vi "TEST AMI 430.vi"() -> ()   [LabVIEW 2017]
uses:
  magneticField.ctl
  Status AMI.ctl
  AMI 430_Hardware_Module.ctl
  commsControl.ctl
panel:
  out "state X":T1=1 items=["Unknown", "RAMPING to target field/current", "HOLDING at the target field/current", "PAUSED", "Ramping in MANUAL UP mode", "Ramping in MANUAL DOWN mode", "ZEROING CURRENT (in progress)", "Quench detected", "At ZERO current", "Heating persistent switch", "Cooling persistent switch", "External Rampdown active"]
  out "state Y":T1=1 items=["Unknown", "RAMPING to target field/current", "HOLDING at the target field/current", "PAUSED", "Ramping in MANUAL UP mode", "Ramping in MANUAL DOWN mode", "ZEROING CURRENT (in progress)", "Quench detected", "At ZERO current", "Heating persistent switch", "Cooling persistent switch", "External Rampdown active"]
  out "state Z":T1=1 items=["Unknown", "RAMPING to target field/current", "HOLDING at the target field/current", "PAUSED", "Ramping in MANUAL UP mode", "Ramping in MANUAL DOWN mode", "ZEROING CURRENT (in progress)", "Quench detected", "At ZERO current", "Heating persistent switch", "Cooling persistent switch", "External Rampdown active"]
  out "Z field":dbl format="%.6f"
  out "Y field":dbl format="%.6f"
  out "X field":dbl format="%.6f"
  in  "RAMPING Z":bool
  in  "RAMPING Y":bool
  in  "RAMPING X":bool
  in  "SET X":bool
  in  "SET Z":bool
  in  "SET Y":bool
  in  "Settings X":T2={"magneticFieldUnits"=1, "rampRateUnits"=1, "rampRate"=0.0, "targetField"=0.0, "rampingMode"=1} {"rampingMode" items=["RAMP", "PAUSE", "MANUAL UP", "MANUAL DOWN", "ZERO"]; "targetField" format="%.3f"; "rampRate" format="%.3f"; "rampRateUnits" items=["Per SECOND", "Per MINUTE"]; "magneticFieldUnits" items=["KGauss", "Tesla"]}
  in  "Settings Z":T2={"magneticFieldUnits"=1, "rampRateUnits"=1, "rampRate"=0.0, "targetField"=0.0, "rampingMode"=1} {"rampingMode" items=["RAMP", "PAUSE", "MANUAL UP", "MANUAL DOWN", "ZERO"]; "targetField" format="%.3f"; "rampRate" format="%.3f"; "rampRateUnits" items=["Per SECOND", "Per MINUTE"]; "magneticFieldUnits" items=["KGauss", "Tesla"]}
  in  "Settings Y":T2={"magneticFieldUnits"=1, "rampRateUnits"=1, "rampRate"=0.0, "targetField"=0.0, "rampingMode"=1} {"rampingMode" items=["RAMP", "PAUSE", "MANUAL UP", "MANUAL DOWN", "ZERO"]; "targetField" format="%.3f"; "rampRate" format="%.3f"; "rampRateUnits" items=["Per SECOND", "Per MINUTE"]; "magneticFieldUnits" items=["KGauss", "Tesla"]}
  out "Waveform Chart":T3(graph)
  out "error out":errorcluster
  in  "stop":bool
  # "AMI 430 MAGNETIC FIELD SYSTEM TEST PANEL"
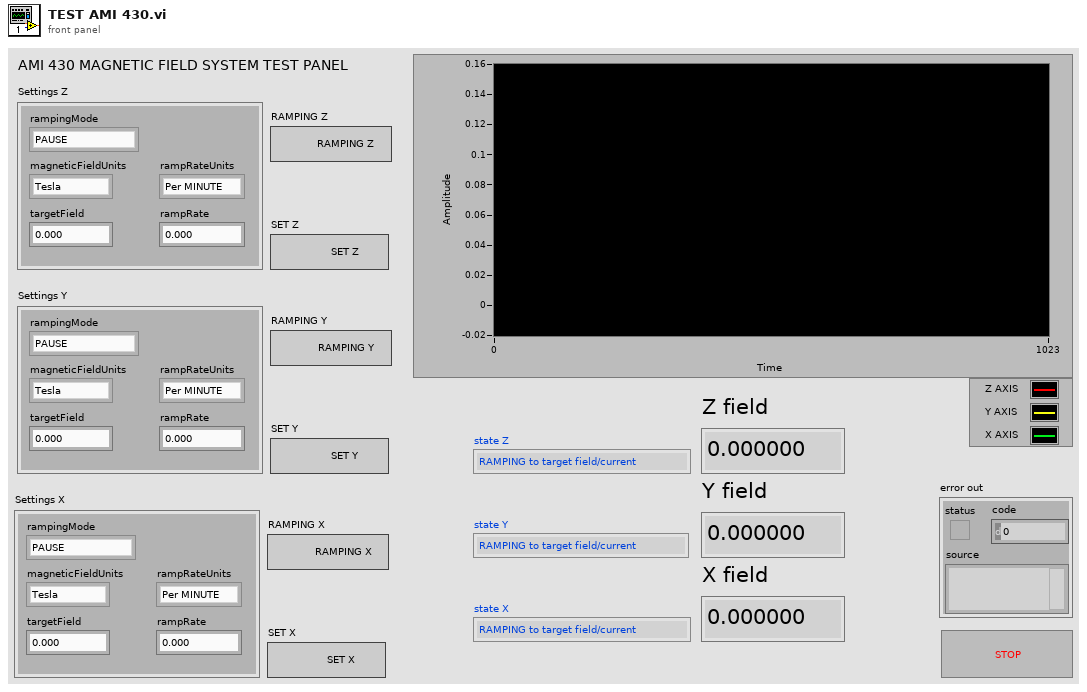
[diagram p1: front panel]
types:
  T1 = typedef "Status AMI.ctl" = u16
  T2 = typedef "magneticField.ctl" = cluster{"magneticFieldUnits":u16, "rampRateUnits":u16, "rampRate":dbl, "targetField":dbl, "rampingMode":u16}
  T3 = cluster{"magneticField":dbl, "magneticField":dbl, "magneticField":dbl}
  T4 = typedef "AMI 430_Hardware_Module.ctl" = enum16{"INICIALIZAR", "SET UNIDADES CAMPO", "SET UNIDADES RAMPA", "SET CAMPO", "SET  RAMPA", "SET RAMPING MODE", "READ CAMPO", "STATUS", "SHUTDOWN"}
  T5 = typedef "commsControl.ctl" = cluster{"connection ID":refnum<k5>, "IP":string, "Active Comm Interface":u16, "Serial Port":refnum<visa-resource-name>, "Programmer Type":u16, "connection ID":refnum<k5>, "output cluster":cluster{"GPIB address":i16, "GPIB bus":i16}}
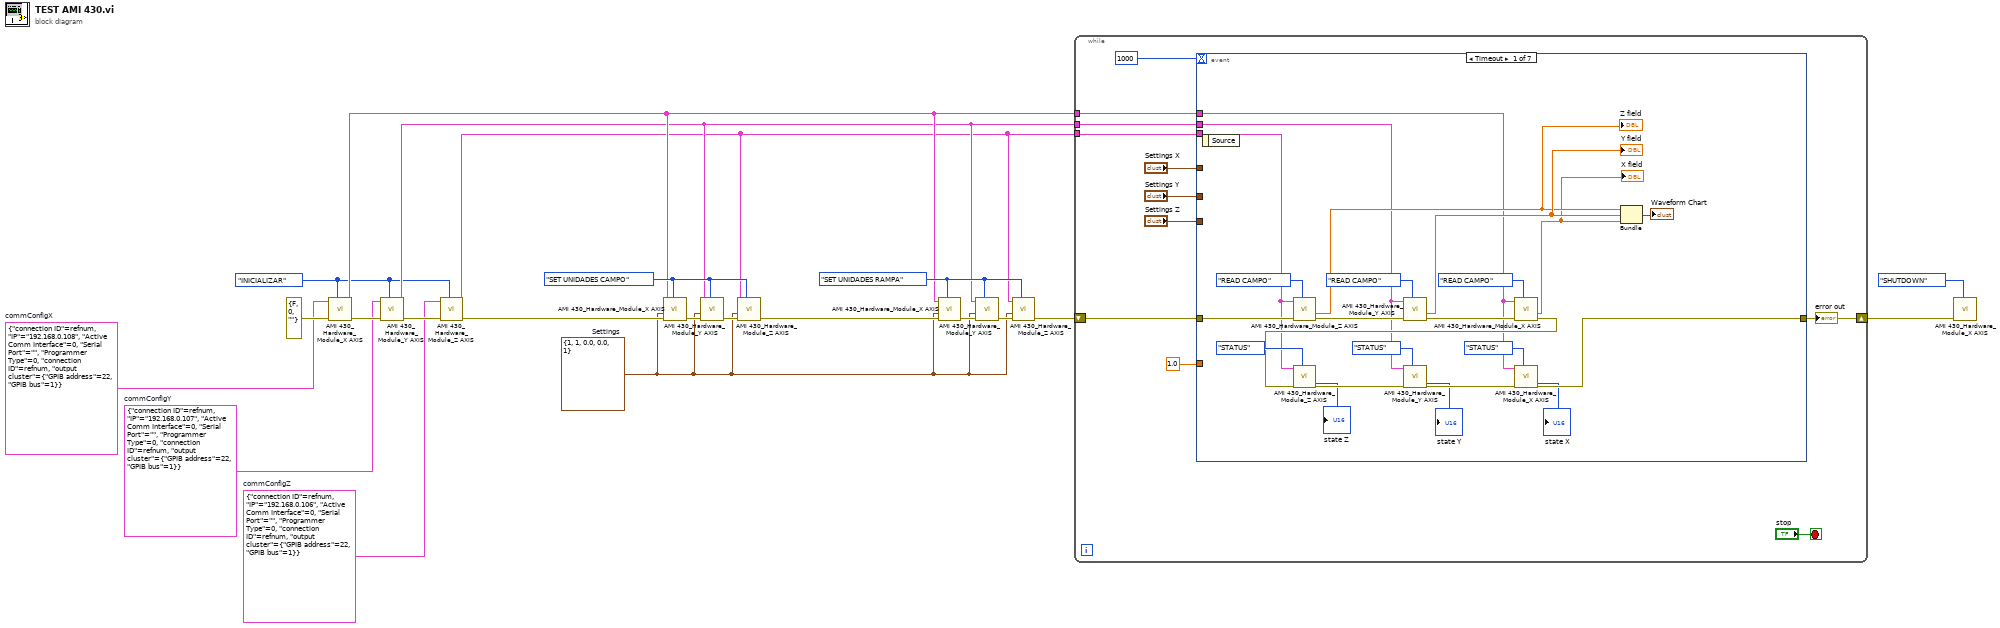
[diagram p0: block diagram]
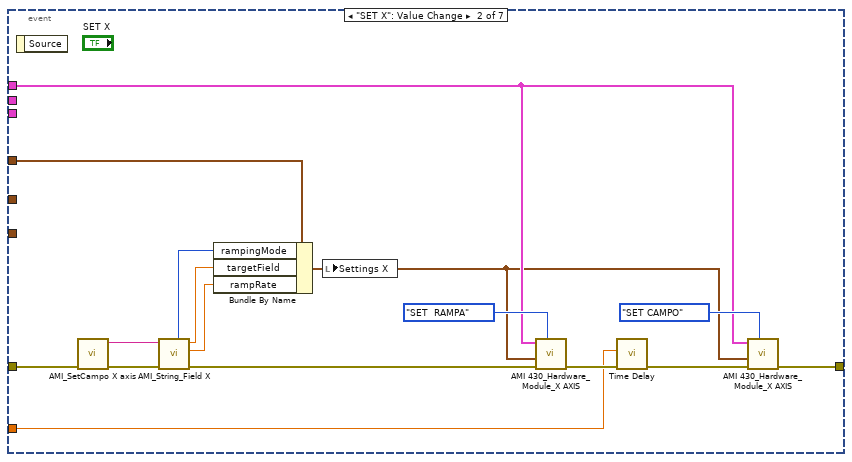
[diagram p2: hidden frame]
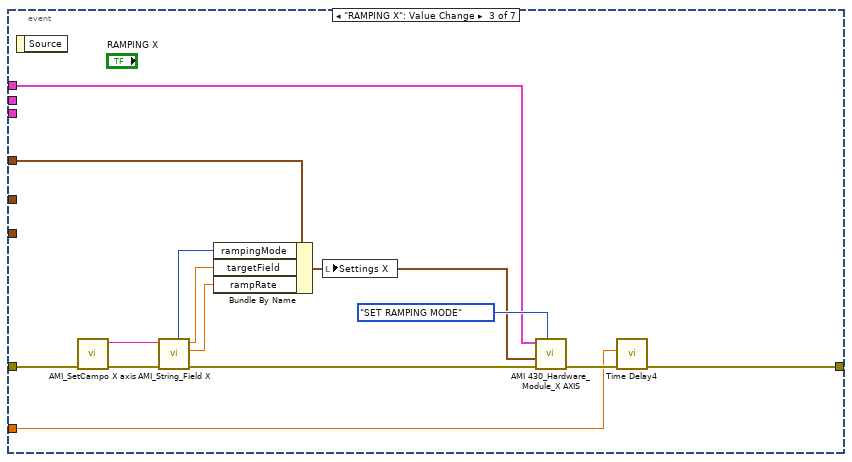
[diagram p3: hidden frame]
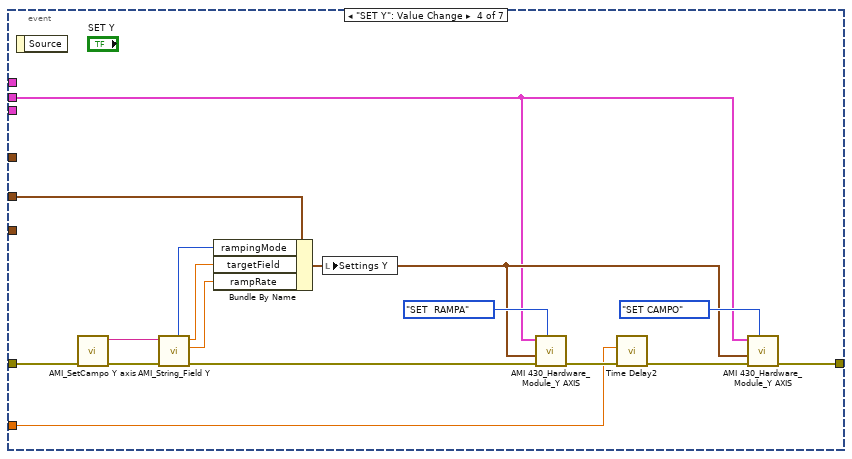
[diagram p4: hidden frame]
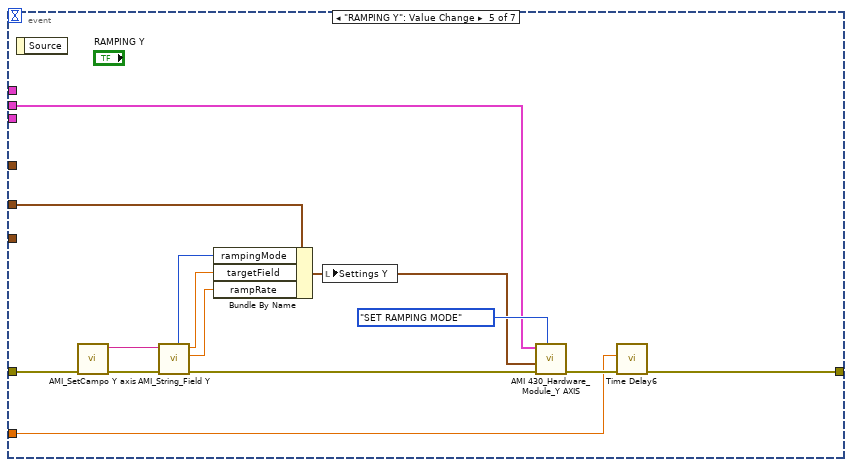
[diagram p5: hidden frame]
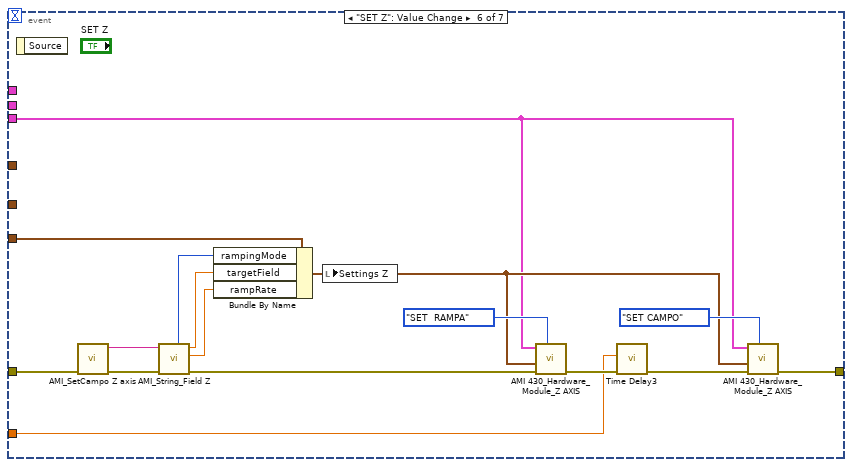
[diagram p6: hidden frame]
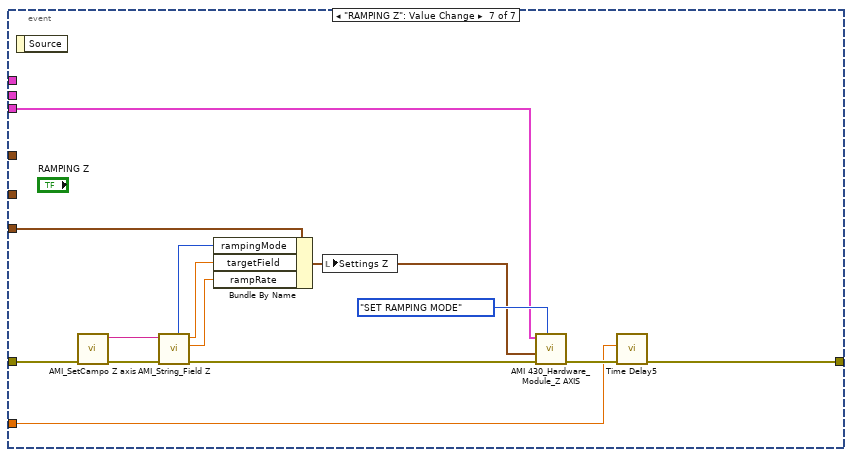
[diagram p7: hidden frame]
diagram:
  w8 = T2 {"magneticFieldUnits"=1, "rampRateUnits"=1, "rampRate"=0.0, "targetField"=0.0, "rampingMode"=1}  # Settings
  w13 = AMI_430_Hardware_Module."SET UNIDADES RAMPA" ("Command")
  w14 = AMI_430_Hardware_Module."SET UNIDADES CAMPO" ("Command")
  w5 = T5 {"connection ID"=refnum, "IP"="192.168.0.106", "Active Comm Interface"=0, "Serial Port"="", "Programmer Type"=0, "connection ID"=refnum, "output cluster"={"GPIB address"=22, "GPIB bus"=1}}  # commConfigZ
  w6 = T5 {"connection ID"=refnum, "IP"="192.168.0.107", "Active Comm Interface"=0, "Serial Port"="", "Programmer Type"=0, "connection ID"=refnum, "output cluster"={"GPIB address"=22, "GPIB bus"=1}}  # commConfigY
  w7 = T5 {"connection ID"=refnum, "IP"="192.168.0.108", "Active Comm Interface"=0, "Serial Port"="", "Programmer Type"=0, "connection ID"=refnum, "output cluster"={"GPIB address"=22, "GPIB bus"=1}}  # commConfigX
  w1 = AMI_430_Hardware_Module."INICIALIZAR" ("Command")
  n1 = call "AMI 430_Hardware_Module_X AXIS.vi"("Command"=w1, "error in (no error)"=errorcluster {"status"=FALSE, "code"=0, "source"=""}, "Comm Config In"=w7) -> ("error out"=w18:errorcluster, "Comm Config Out"=w4:T5)  [unwired: 4 in, 3 out]
  n2 = call "AMI 430_Hardware_Module_Y AXIS.vi"("Command"=w1, "error in (no error)"=w18, "Comm Config In"=w6) -> ("error out"=w19:errorcluster, "Comm Config Out"=w3:T5)  [unwired: 4 in, 3 out]
  n3 = call "AMI 430_Hardware_Module_Z AXIS.vi"("Command"=w1, "error in (no error)"=w19, "Comm Config In"=w5) -> ("error out"=w15:errorcluster, "Comm Config Out"=w2:T5)  [unwired: 4 in, 3 out]
  n4 = call "AMI 430_Hardware_Module_X AXIS.vi"("Command"=w14, "error in (no error)"=w15, "Settings"=w8, "Comm Config In"=w4) -> ("error out"=w17:errorcluster)  [unwired: 3 in, 4 out]
  n5 = call "AMI 430_Hardware_Module_Y AXIS.vi"("Command"=w14, "error in (no error)"=w17, "Settings"=w8, "Comm Config In"=w3) -> ("error out"=w16:errorcluster)  [unwired: 3 in, 4 out]
  n6 = call "AMI 430_Hardware_Module_Z AXIS.vi"("Command"=w14, "error in (no error)"=w16, "Settings"=w8, "Comm Config In"=w2) -> ("error out"=w10:errorcluster)  [unwired: 3 in, 4 out]
  n7 = call "AMI 430_Hardware_Module_X AXIS.vi"("Command"=w13, "error in (no error)"=w10, "Settings"=w8, "Comm Config In"=w4) -> ("error out"=w12:errorcluster)  [unwired: 3 in, 4 out]
  n8 = call "AMI 430_Hardware_Module_Y AXIS.vi"("Command"=w13, "error in (no error)"=w12, "Settings"=w8, "Comm Config In"=w3) -> ("error out"=w11:errorcluster)  [unwired: 3 in, 4 out]
  n9 = call "AMI 430_Hardware_Module_Z AXIS.vi"("Command"=w13, "error in (no error)"=w11, "Settings"=w8, "Comm Config In"=w2) -> ("error out"=w9:errorcluster)  [unwired: 3 in, 4 out]
  n10 = while {
    shift-right: [w31] -> w21
    shift-left: w9 -> [w32]
    tunnel: w4 -> [w29]
    tunnel: w3 -> [w28]
    tunnel: w2 -> [w27]
    stop <- "stop" stop-if-true
    n11 = event shown="[0] Timeout" {
      selector: _ -> [_ _ _ _ _ _ _]
      dyn-events: _ -> [_ _ _ _ _ _ _]
      timeout: 1000 -> [_ _ _ _ _ _ _]
      tunnel: w32 -> [w55 w70 w84 w100 w114 w130 w144]
      tunnel: [w42 w61 w74 w91 w104 w121 w134] -> w31
      tunnel: w29 -> [w37 w59 w76 _ _ _ _]
      tunnel: w28 -> [w38 _ _ w87 w103 _ _]
      tunnel: w27 -> [w39 _ _ _ _ w117 w133]
      tunnel: 1.0 ("Delay Time (s)") -> [_ w63 w77 w93 w107 w123 w137]
      tunnel: "Settings X" -> [_ w57 w73 _ _ _ _]
      tunnel: "Settings Z" -> [_ _ _ _ _ w118 w135]
      tunnel: "Settings Y" -> [_ _ _ w88 w105 _ _]
      event Timeout {
        n12 = event-data() -> ()  [unwired: 1 in, 1 out]
        n13 = call "AMI 430_Hardware_Module_Z AXIS.vi"("Command"=AMI_430_Hardware_Module."READ CAMPO", "error in (no error)"=w55, "Comm Config In"=w39) -> ("error out"=w51:errorcluster, "magneticField"=w48:dbl)  [unwired: 4 in, 3 out]
        "Z field" <- w48
        n14 = call "AMI 430_Hardware_Module_Y AXIS.vi"("Command"=AMI_430_Hardware_Module."READ CAMPO", "error in (no error)"=w51, "Comm Config In"=w38) -> ("error out"=w52:errorcluster, "magneticField"=w49:dbl)  [unwired: 4 in, 3 out]
        "Y field" <- w49
        n15 = call "AMI 430_Hardware_Module_X AXIS.vi"("Command"=AMI_430_Hardware_Module."READ CAMPO", "error in (no error)"=w52, "Comm Config In"=w37) -> ("error out"=w43:errorcluster, "magneticField"=w47:dbl)  [unwired: 4 in, 3 out]
        "X field" <- w47
        n16 = call "AMI 430_Hardware_Module_Z AXIS.vi"("Command"=AMI_430_Hardware_Module."STATUS", "error in (no error)"=w43, "Comm Config In"=w39) -> ("error out"=w40:errorcluster, "state"=→"state Z":T1)  [unwired: 4 in, 3 out]
        n17 = call "AMI 430_Hardware_Module_Y AXIS.vi"("Command"=AMI_430_Hardware_Module."STATUS", "error in (no error)"=w40, "Comm Config In"=w38) -> ("error out"=w41:errorcluster, "state"=→"state Y":T1)  [unwired: 4 in, 3 out]
        n18 = call "AMI 430_Hardware_Module_X AXIS.vi"("Command"=AMI_430_Hardware_Module."STATUS", "error in (no error)"=w41, "Comm Config In"=w37) -> ("error out"=w42:errorcluster, "state"=→"state X":T1)  [unwired: 4 in, 3 out]
        n19 = Bundle("magneticField"=w48, "magneticField"=w49, "magneticField"=w47) -> (→"Waveform Chart":T3)  [unwired: 1 in]
      }
      event "SET X": Value Change {
        n20 = event-data() -> ()  [unwired: 1 in, 1 out]
        n21 = call "AMI_SetCampo X axis.vi"("error in (no error)"=w70) -> ("error out"=w66:errorcluster, "resulting string X"=w67:string)  [unwired: 7 in]
        n22 = call "AMI_String_Field X.vi"("error in (no error)"=w66, "String"=w67) -> ("error out"=w65:errorcluster, "X Rate"=w68:dbl, "X Field"=w69:dbl, "X Modo Rampa"=w64:u16)  [unwired: 5 in, 1 out]
        n23 = Bundle By Name(cluster=w57, "rampingMode"=w64, "targetField"=w69, "rampRate"=w68) -> (w58:T2)
        n24 = local write "Settings X"(w58) -> ()
        n25 = call "AMI 430_Hardware_Module_X AXIS.vi"("Command"=AMI_430_Hardware_Module."SET  RAMPA", "error in (no error)"=w65, "Settings"=w58, "Comm Config In"=w59) -> ("error out"=w72:errorcluster)  [unwired: 3 in, 4 out]
        n26 = call "Time Delay"("error in (no error)"=w72, "Delay Time (s)"=w63) -> ("error out"=w62:errorcluster)  [unwired: 9 in]
        n27 = call "AMI 430_Hardware_Module_X AXIS.vi"("Command"=AMI_430_Hardware_Module."SET CAMPO", "error in (no error)"=w62, "Settings"=w58, "Comm Config In"=w59) -> ("error out"=w61:errorcluster)  [unwired: 3 in, 4 out]
      }
      event "RAMPING X": Value Change {
        n28 = event-data() -> ()  [unwired: 1 in, 1 out]
        n29 = call "AMI_SetCampo X axis.vi"("error in (no error)"=w84) -> ("error out"=w80:errorcluster, "resulting string X"=w81:string)  [unwired: 7 in]
        n30 = call "AMI_String_Field X.vi"("error in (no error)"=w80, "String"=w81) -> ("error out"=w79:errorcluster, "X Rate"=w82:dbl, "X Field"=w83:dbl, "X Modo Rampa"=w78:u16)  [unwired: 5 in, 1 out]
        n31 = Bundle By Name(cluster=w73, "rampingMode"=w78, "targetField"=w83, "rampRate"=w82) -> (w75:T2)
        n32 = local write "Settings X"(w75) -> ()
        n33 = call "AMI 430_Hardware_Module_X AXIS.vi"("Command"=AMI_430_Hardware_Module."SET RAMPING MODE", "error in (no error)"=w79, "Settings"=w75, "Comm Config In"=w76) -> ("error out"=w86:errorcluster)  [unwired: 3 in, 4 out]
        n34 = call "Time Delay4"("error in (no error)"=w86, "Delay Time (s)"=w77) -> ("error out"=w74:errorcluster)  [unwired: 9 in]
      }
      event "SET Y": Value Change {
        n35 = event-data() -> ()  [unwired: 1 in, 1 out]
        n36 = call "AMI_SetCampo Y axis.vi"("error in (no error)"=w100) -> ("error out"=w96:errorcluster, "resulting string Y"=w97:string)  [unwired: 7 in]
        n37 = call "AMI_String_Field Y.vi"("error in (no error)"=w96, "String"=w97) -> ("error out"=w95:errorcluster, "Y Rate"=w98:dbl, "Y Field"=w99:dbl, "Y Modo Rampa"=w94:u16)  [unwired: 5 in, 1 out]
        n38 = Bundle By Name(cluster=w88, "rampingMode"=w94, "targetField"=w99, "rampRate"=w98) -> (w89:T2)
        n39 = local write "Settings Y"(w89) -> ()
        n40 = call "AMI 430_Hardware_Module_Y AXIS.vi"("Command"=AMI_430_Hardware_Module."SET  RAMPA", "error in (no error)"=w95, "Settings"=w89, "Comm Config In"=w87) -> ("error out"=w102:errorcluster)  [unwired: 3 in, 4 out]
        n41 = call "Time Delay2"("error in (no error)"=w102, "Delay Time (s)"=w93) -> ("error out"=w92:errorcluster)  [unwired: 9 in]
        n42 = call "AMI 430_Hardware_Module_Y AXIS.vi"("Command"=AMI_430_Hardware_Module."SET CAMPO", "error in (no error)"=w92, "Settings"=w89, "Comm Config In"=w87) -> ("error out"=w91:errorcluster)  [unwired: 3 in, 4 out]
      }
      event "RAMPING Y": Value Change {
        n43 = event-data() -> ()  [unwired: 1 in, 1 out]
        n44 = call "AMI_SetCampo Y axis.vi"("error in (no error)"=w114) -> ("error out"=w110:errorcluster, "resulting string Y"=w111:string)  [unwired: 7 in]
        n45 = call "AMI_String_Field Y.vi"("error in (no error)"=w110, "String"=w111) -> ("error out"=w109:errorcluster, "Y Rate"=w112:dbl, "Y Field"=w113:dbl, "Y Modo Rampa"=w108:u16)  [unwired: 5 in, 1 out]
        n46 = Bundle By Name(cluster=w105, "rampingMode"=w108, "targetField"=w113, "rampRate"=w112) -> (w106:T2)
        n47 = local write "Settings Y"(w106) -> ()
        n48 = call "AMI 430_Hardware_Module_Y AXIS.vi"("Command"=AMI_430_Hardware_Module."SET RAMPING MODE", "error in (no error)"=w109, "Settings"=w106, "Comm Config In"=w103) -> ("error out"=w116:errorcluster)  [unwired: 3 in, 4 out]
        n49 = call "Time Delay6"("error in (no error)"=w116, "Delay Time (s)"=w107) -> ("error out"=w104:errorcluster)  [unwired: 9 in]
      }
      event "SET Z": Value Change {
        n50 = event-data() -> ()  [unwired: 1 in, 1 out]
        n51 = call "AMI_SetCampo Z axis.vi"("error in (no error)"=w130) -> ("error out"=w126:errorcluster, "resulting string Z"=w127:string)  [unwired: 7 in]
        n52 = call "AMI_String_Field Z.vi"("error in (no error)"=w126, "String"=w127) -> ("error out"=w125:errorcluster, "Z Rate"=w128:dbl, "Z Field"=w129:dbl, "Z Modo Rampa"=w124:u16)  [unwired: 5 in, 1 out]
        n53 = Bundle By Name(cluster=w118, "rampingMode"=w124, "targetField"=w129, "rampRate"=w128) -> (w119:T2)
        n54 = local write "Settings Z"(w119) -> ()
        n55 = call "AMI 430_Hardware_Module_Z AXIS.vi"("Command"=AMI_430_Hardware_Module."SET  RAMPA", "error in (no error)"=w125, "Settings"=w119, "Comm Config In"=w117) -> ("error out"=w132:errorcluster)  [unwired: 3 in, 4 out]
        n56 = call "Time Delay3"("error in (no error)"=w132, "Delay Time (s)"=w123) -> ("error out"=w122:errorcluster)  [unwired: 9 in]
        n57 = call "AMI 430_Hardware_Module_Z AXIS.vi"("Command"=AMI_430_Hardware_Module."SET CAMPO", "error in (no error)"=w122, "Settings"=w119, "Comm Config In"=w117) -> ("error out"=w121:errorcluster)  [unwired: 3 in, 4 out]
      }
      event "RAMPING Z": Value Change {
        n58 = event-data() -> ()  [unwired: 1 in, 1 out]
        n59 = call "AMI_SetCampo Z axis.vi"("error in (no error)"=w144) -> ("error out"=w140:errorcluster, "resulting string Z"=w141:string)  [unwired: 7 in]
        n60 = call "AMI_String_Field Z.vi"("error in (no error)"=w140, "String"=w141) -> ("error out"=w139:errorcluster, "Z Rate"=w142:dbl, "Z Field"=w143:dbl, "Z Modo Rampa"=w138:u16)  [unwired: 5 in, 1 out]
        n61 = Bundle By Name(cluster=w135, "rampingMode"=w138, "targetField"=w143, "rampRate"=w142) -> (w136:T2)
        n62 = local write "Settings Z"(w136) -> ()
        n63 = call "AMI 430_Hardware_Module_Z AXIS.vi"("Command"=AMI_430_Hardware_Module."SET RAMPING MODE", "error in (no error)"=w139, "Settings"=w136, "Comm Config In"=w133) -> ("error out"=w146:errorcluster)  [unwired: 3 in, 4 out]
        n64 = call "Time Delay5"("error in (no error)"=w146, "Delay Time (s)"=w137) -> ("error out"=w134:errorcluster)  [unwired: 9 in]
      }
    }
    "error out" <- w31
  }
  n65 = call "AMI 430_Hardware_Module_X AXIS.vi"("Command"=AMI_430_Hardware_Module."SHUTDOWN", "error in (no error)"=w21) -> ()  [unwired: 5 in, 5 out]
